vi "Main.vi"() -> ()   [LabVIEW 2014]
doc: "The Reaper Controller\n\nMarcin Twardak - twardakm@gmail.com\nLeszek Walulik\nJarosław Woźniak"
uses:
  Controls/Connection Configuration.ctl
  Controls/Controllers Clusters/Normal Operation Control Cluster.ctl
  Controls/Controllers.ctl
  Controls/Controllers Clusters/General Control Cluster.ctl
  Controls/Controllers Clusters/Game Pad Indicator Cluster.ctl
  Controls/Controllers Clusters/Game Pad Control Cluster.ctl
  Controls/Controllers Clusters/Mouse Control Cluster.ctl
  Controls/Queue Commands.ctl
  Controls/User Events Commands.ctl
  Controls/Connection Status.ctl
  Controls/User Help.ctl
  Controls/Configuration Files.ctl
  Controls/Simple Connection Settings Cluster.ctl
  <vilib>/Utility/miscctls.llb/LVBoundsTypeDef.ctl
  <vilib>/event_ctls.llb/usereventprio.ctl
  SubVIs/Convert From XML Configuration Files - Polymorphic/Simple Connection Settings Polymorphic.vi
  SubVIs/Convert From XML Configuration Files - Polymorphic/General Control Settings Polymporhic.vi
panel:
  in  "Normal Operation\nControl Cluster":T1 {"Game Pad Control Cluster"."Steering Wheel [Test]" scale=-100.0..100.0; "Game Pad Control Cluster"."Speed [Test]" scale=-100.0..100.0; "Game Pad Indicator Cluster"."Steering Wheel [%]" scale=-100.0..100.0; "Game Pad Indicator Cluster"."Speed" scale=0.0..100.0; "General Control Cluster"."Max Speed" max=100 step=5 scale=0.0..100.0}
  in  "Connection Conf\nCluster":T7
  out "User Help":string
  in  "Stop Button":bool
  # "THE REAPER"
  # "[Ctrl + Num] to switch"
  # "Mouse Controller"
  # "Game Pad Controller"
  # "Connection Configuration"
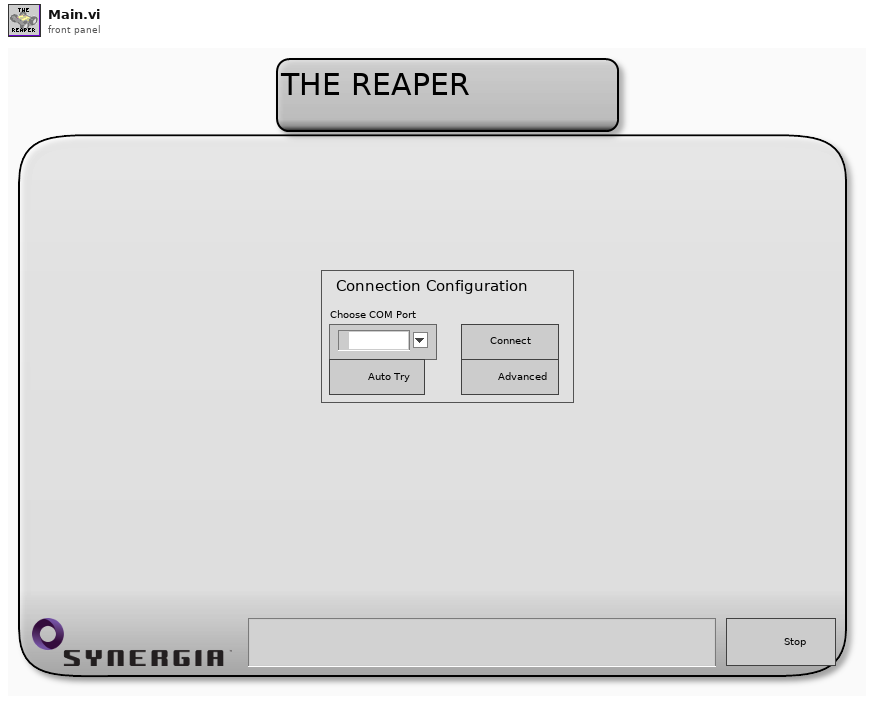
[diagram p1: front panel]
types:
  T1 = typedef "Normal Operation Control Cluster.ctl" = cluster{"Disconnect Button":bool, "Control Type":T2, "General Control Cluster":T3, "Game Pad Indicator Cluster":T4, "Game Pad Control Cluster":T5, "Mouse Control Cluster":T6}
  T2 = typedef "Controllers.ctl" = enum16{"Turned off", "Keyboard", "Mouse", "Pad", "Autonomous"}
  T3 = typedef "General Control Cluster.ctl" = cluster{"Max Speed":u8}
  T4 = typedef "Game Pad Indicator Cluster.ctl" = cluster{"Speed":u8, "Motor On?":bool, "Steering Wheel [%]":i8}
  T5 = typedef "Game Pad Control Cluster.ctl" = cluster{"Advanced Settings":bool, "Speed [Test]":i8, "Steering Wheel [Test]":i8, "Motor On [Test]":bool}
  T6 = typedef "Mouse Control Cluster.ctl" = cluster{"Mouse Controller":picture}
  T7 = typedef "Connection Configuration.ctl" = cluster{"Choose COM Port":refnum<visa-resource-name>, "Connect Button":bool, "Advanced Button":bool, "Auto Try Button":bool}
  T8 = typedef "Connection Status.ctl" = enum16{"Disconnected", "Connected"}
  T9 = typedef "User Events Commands.ctl" = enum16{"Consumer Error", "Stop App"}
  T10 = typedef "Queue Commands.ctl" = enum16{"Init", "Close App", "Producer Error", "Connect", "Try Auto Connect", "Is Connected?", "Advanced Connection Settings", "Disconnect", "Change Control Mode", "Stop Turn Off", "Start Turn Off", "Stop Keyboard", "Start Keyboard", "Stop Mouse", "Start Mouse", "Mouse", "Stop Pad", "Start Pad", "Pad", "Pad Advanced Settings", "Stop Autonomous", "Start Autonomous"}
  T11 = typedef "Configuration Files.ctl" = string
  T12 = typedef "Simple Connection Settings Cluster.ctl" = refnum<visa-resource-name>
  T13 = typedef "User Help.ctl" = enum16{"The Reaper Controller says hello!\nFirst you should establish connection with The Reaper.", "Connection established! Choose control mode.", "Something went wrong. Try another COM port.", "Disconnected. Do you want to connect again?", "Controls turned off", "Keyboard Mode", "Mouse Mode", "Pad Mode", "Autonomous Mode", "Unknown Operation occured", "Please connect before choosing control type!", "Settings available only if disconnected.", "Settings updated."}
  T14 = cluster{"Width":u16, "Style":enum32{"Solid", "Dash", "Dot", "DashDot", "DashDotDot"}}
  T15 = typedef "LVBoundsTypeDef.ctl" = cluster{"Width":u32, "Height":u32}
  T16 = typedef "usereventprio.ctl" = enum32{"high priority", "normal priority"}
  T17 = typedef "LVMouseTypeDef.ctl" = cluster{"Mouse Position":cluster{"X":i32, "Y":i32}, "Mouse Modifiers":cluster{"Button Down":bool, "Shift Mod":bool, "Menu Mod":bool, "Option Mod":bool}}
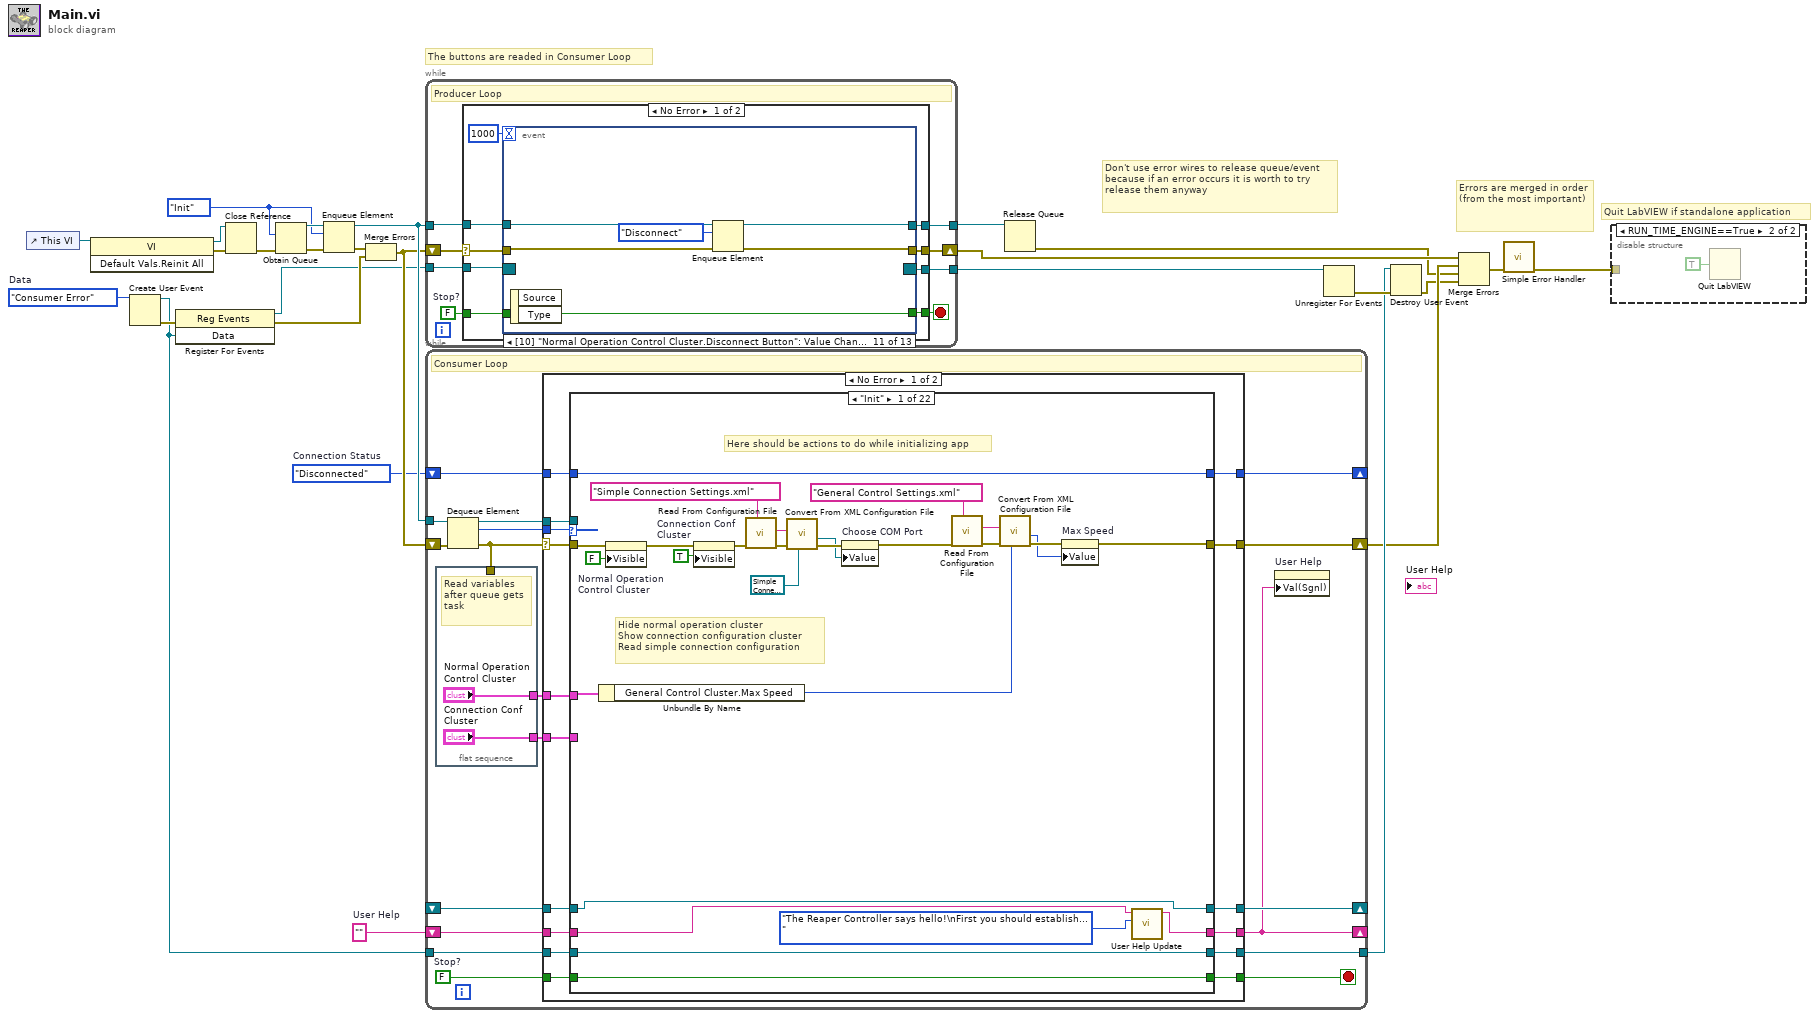
[diagram p0: block diagram]
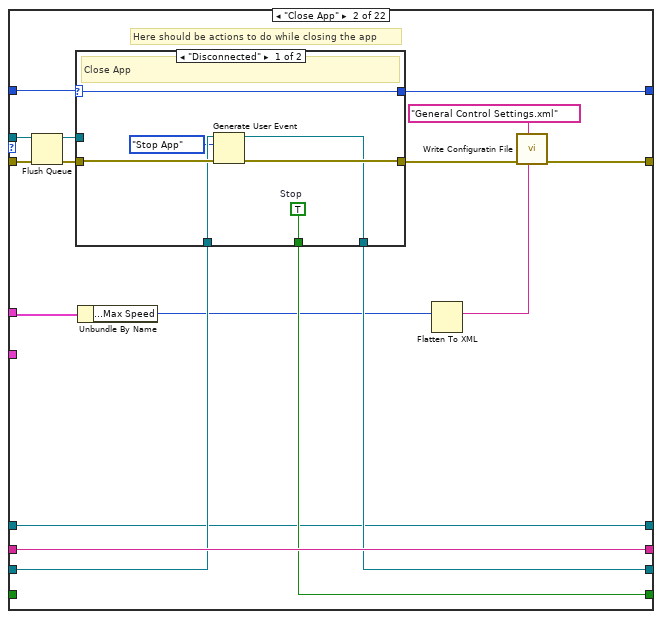
[diagram p3: hidden frame]
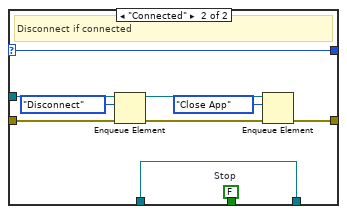
[diagram p4: hidden frame]
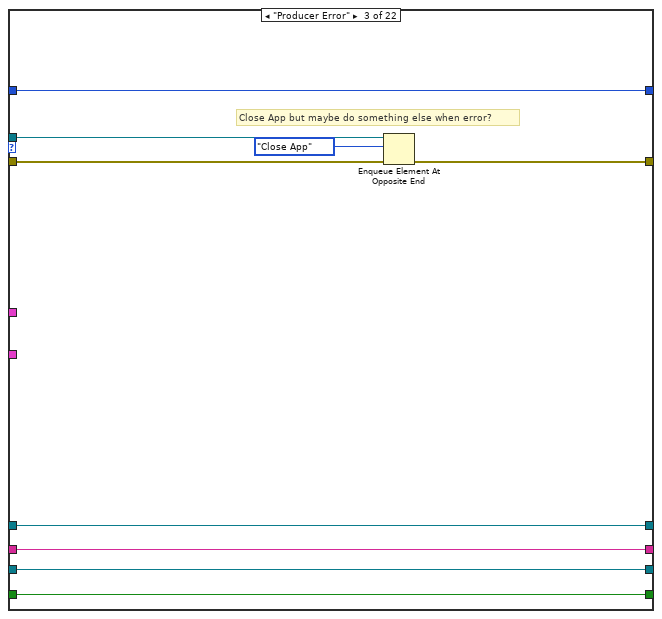
[diagram p5: hidden frame]
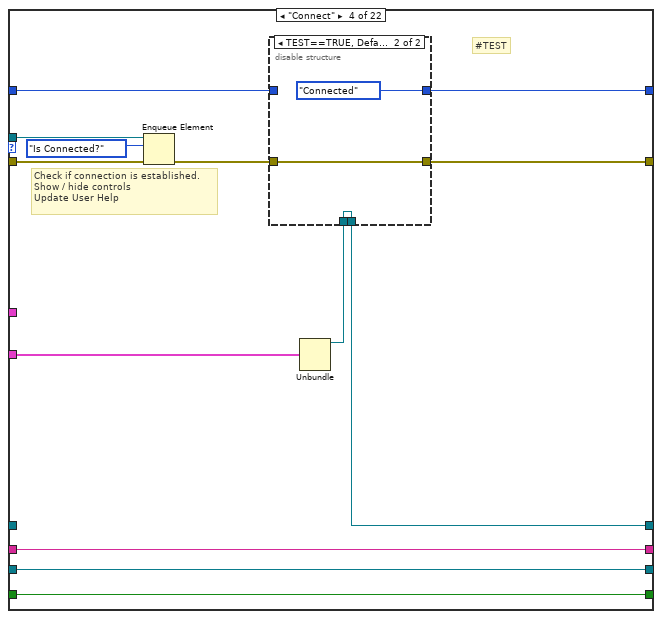
[diagram p6: hidden frame]
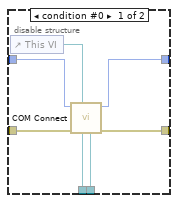
[diagram p7: hidden frame]
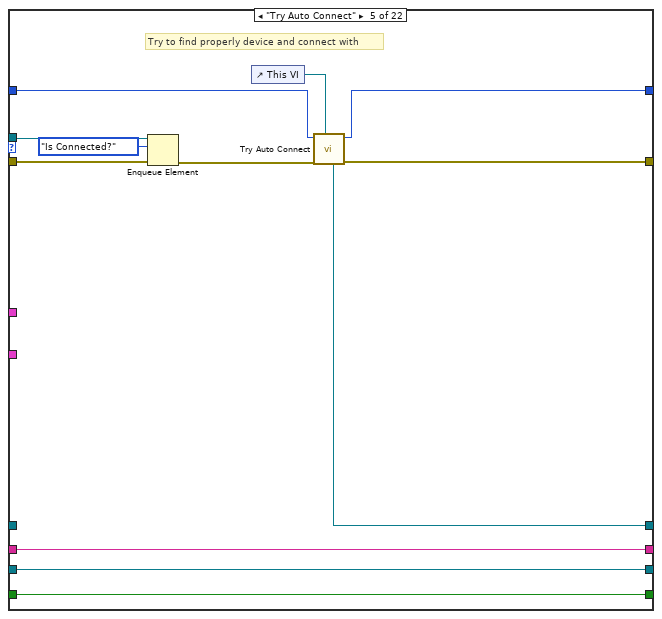
[diagram p8: hidden frame]
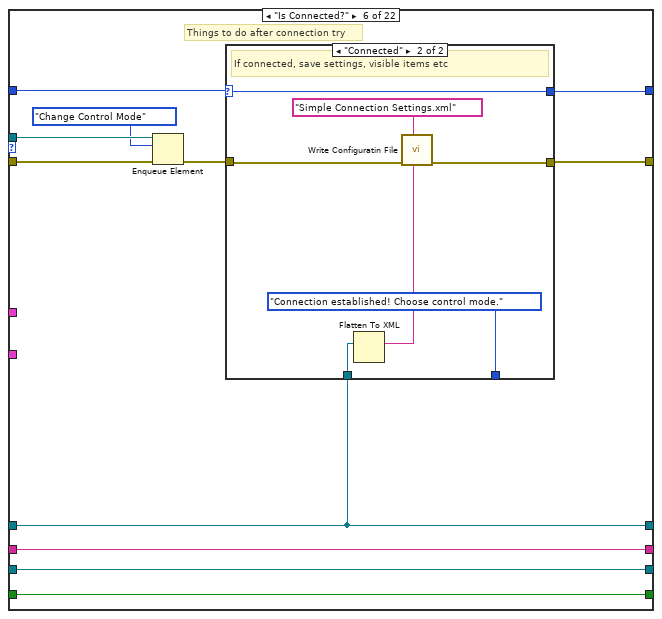
[diagram p9: hidden frame]
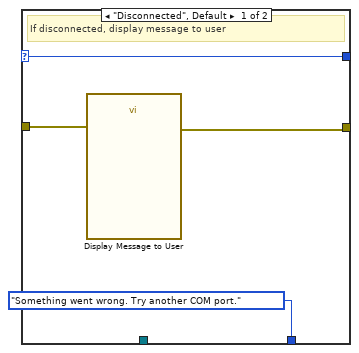
[diagram p10: hidden frame]
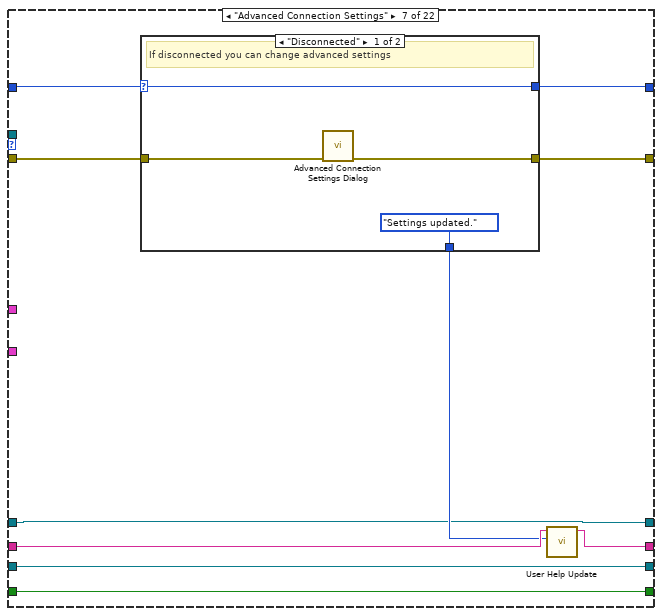
[diagram p11: hidden frame]
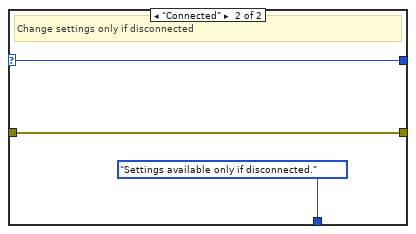
[diagram p12: hidden frame]
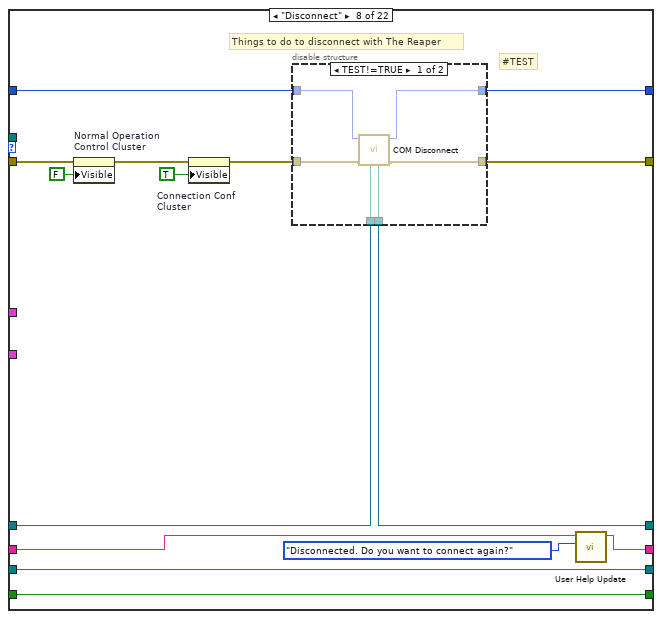
[diagram p13: hidden frame]
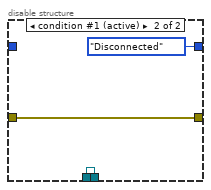
[diagram p14: hidden frame]
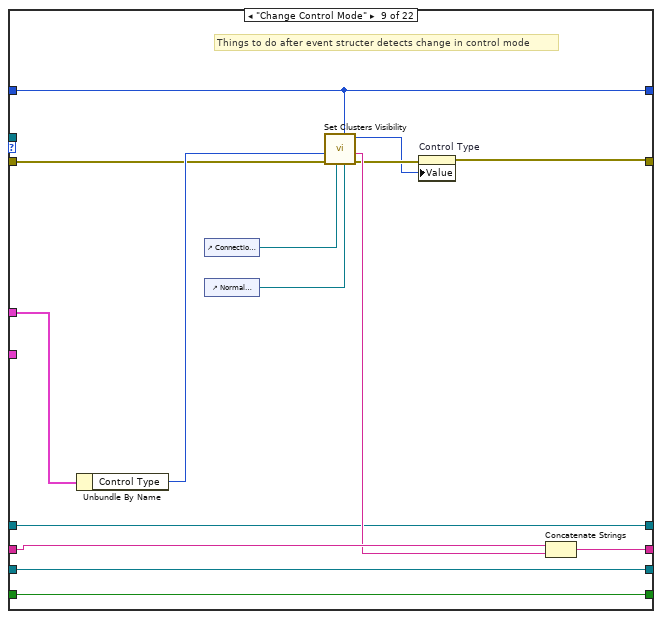
[diagram p15: hidden frame]
diagram:
  w1 = Connection_Status."Disconnected"  # Connection Status
  w3 = ""  # User Help
  w20 = User_Events_Commands."Consumer Error"  # Data
  w2 = Queue_Commands."Init"
  # "The buttons are readed in Consumer Loop"
  # "Quit LabVIEW if standalone application"
  # "Don't use error wires to release queue/event  because if an error occurs it is worth to try release them anyway"
  # "Errors are merged in order (from the most important)"
  n1 = control-ref of="This VI"() -> (w27:refnum<vi>)
  n2 = invoke class="VI" method="Default Vals.Reinit All"(reference=w27) -> (reference out=w25:refnum<vi>, error out=w26:errorcluster)  [unwired: 2 in, 1 out]
  n3 = Create User Event(user event datatype=w20) -> (user event=w14:refnum<user-event>, error out=w21:errorcluster)  [unwired: 1 in]
  n4 = register-events(error in=w21, w14) -> (reference out=w15:refnum<event-registration>, error out=w18:errorcluster)  [unwired: 1 in]
  n5 = Close Reference(reference=w25, error in (no error)=w26) -> (error out=w24:errorcluster)
  n6 = Obtain Queue(element data type=w2, error in (no error)=w24) -> (queue out=w22:refnum<queue>, error out=w23:errorcluster)  [unwired: 3 in, 1 out]
  n7 = Enqueue Element(queue=w22, element=w2, error in (no error)=w23) -> (queue out=w17:refnum<queue>, error out=w19:errorcluster)  [unwired: 1 in, 1 out]
  n8 = Merge Errors(w19, w18) -> (w16:errorcluster)
  n9 = while {
    tunnel: w17 -> [w34]
    shift-right: [w33] -> w9
    shift-left: w16 -> [w35]
    tunnel: w15 -> [w30]
    tunnel: [w29] -> w12
    tunnel: [w28] -> w13
    stop <- w32 stop-if-true
    w31 = FALSE  # Stop?
    # "Producer Loop"
    n10 = case shown="No Error" w35 {
      selector: w35 -> [w41 w176]
      tunnel: w34 -> [w42 w178]
      tunnel: [w40 w175] -> w33
      tunnel: [w37 w174] -> w32
      tunnel: w31 -> [w44 _]
      tunnel: w30 -> [w39 w173]
      tunnel: [w38 w173] -> w29
      tunnel: [w36 w172] -> w28
      frame No Error {
        n11 = event shown="[10] \"Normal Operation Control Cluster.Disconnect Button\": Value Change" {
          selector: w39 -> [_ _ _ _ _ _ _ _ _ _ _ _ _]
          dyn-events: [_ _ _ _ _ _ _ _ _ _ _ _ _] -> w38
          timeout: 1000 -> [_ _ _ _ _ _ _ _ _ _ _ _ _]
          tunnel: w44 -> [w46 _ _ w69 w98 w110 w116 w122 w128 w134 w140 w154 w170]
          tunnel: w42 -> [w45 w53 w58 w67 w96 w109 w115 w119 w127 w133 w139 w153 w169]
          tunnel: w41 -> [w47 w52 w56 w65 w94 w106 w112 w120 w124 w132 w137 w152 w167]
          tunnel: [w47 w51 w55 w64 w93 w105 w113 w121 w125 w131 w136 w144 w166] -> w40
          tunnel: [w46 w50 TRUE ("Stop") w69 w98 w110 w116 w122 w128 w134 w140 w154 w170] -> w37
          tunnel: [w45 w49 w57 w66 w95 w109 w114 w118 w126 w133 w138 w143 w168] -> w36
          event Timeout {
            n12 = event-data() -> ()  [unwired: 1 in, 1 out]
          }
          event "Stop Button": Value Change {
            w50 = FALSE  # Stop
            # "Don't stop\nStop due to User Event"
            n13 = event-data() -> ()  [unwired: 1 in, 1 out]
            n14 = Enqueue Element(queue=w53, element=Queue_Commands."Close App", error in (no error)=w52) -> (queue out=w49:refnum<queue>, error out=w51:errorcluster)  [unwired: 1 in, 1 out]
          }
          event User Event {
            # "User Event is used to catch consumer errors or stop prompt"
            n15 = event-data() -> ("Data"=w59:T9)  [unwired: 1 in]
            n16 = case shown="\"Stop App\"" w59 {
              tunnel: w58 -> [w61 w62]
              tunnel: [w61 w62] -> w57
              tunnel: w56 -> [w60 w63]
              tunnel: [w60 w63] -> w55
              frame "Consumer Error" {
              }
              frame "Stop App" {
              }
            }
          }
          event Menu Selection (User) {
            # "Shortcuts and menus undefined in LabVIEW"
            n17 = event-data() -> ("ItemTag"=w68:string)  [unwired: 1 in]
            n18 = case shown="\"Ctrl_3\"" w68 {
              tunnel: w67 -> [w71 w73 w79 w81 w85 w89]
              tunnel: [w71 w73 w79 w81 w85 w90] -> w66
              tunnel: [w70 w74 w77 w82 w86 w91] -> w64
              tunnel: w65 -> [w70 w75 w78 w83 w87 w92]
              frame Default {
              }
              frame "Ctrl_1" {
                # "Set Keyboard Mode"
                n19 = property on="Control Type" class="Enum (strict)"(error in=w75, "Val(Sgnl)"=Controllers."Keyboard" ("Value (Signaling)")) -> (error out=w74:errorcluster)  [unwired: 1 in, 1 out]
              }
              frame "Ctrl_2" {
                # "Set Mouse Mode"
                n20 = property on="Control Type" class="Enum (strict)"(error in=w78, "Val(Sgnl)"=Controllers."Mouse" ("Value (Signaling)")) -> (error out=w77:errorcluster)  [unwired: 1 in, 1 out]
              }
              frame "Ctrl_3" {
                # "Set Pad Mode"
                n21 = property on="Control Type" class="Enum (strict)"(error in=w83, "Val(Sgnl)"=Controllers."Pad" ("Value (Signaling)")) -> (error out=w82:errorcluster)  [unwired: 1 in, 1 out]
              }
              frame "Ctrl_4" {
                # "Set Autonomous Mode"
                n22 = property on="Control Type" class="Enum (strict)"(error in=w87, "Val(Sgnl)"=Controllers."Autonomous" ("Control Type")) -> (error out=w86:errorcluster)  [unwired: 1 in, 1 out]
              }
              frame "Advanced Settings" {
                # "Advanced Connection Settings"
                n23 = Enqueue Element(queue=w89, element=Queue_Commands."Advanced Connection Settings", error in (no error)=w92) -> (queue out=w90:refnum<queue>, error out=w91:errorcluster)  [unwired: 1 in, 1 out]
              }
            }
          }
          event Key Down {
            # "Other Key activities"
            n24 = event-data() -> ("Char"=w97:i16)  [unwired: 1 in]
            n25 = case shown="32" w97 {
              tunnel: w96 -> [w100 w104]
              tunnel: [w100 w104] -> w95
              tunnel: [w99 w102] -> w93
              tunnel: w94 -> [w99 w103]
              frame Default {
                # "Do nothing"
              }
              frame 32 {
                # "Spacebar - safety button"
                n26 = property on="Control Type" class="Enum (strict)"(error in=w103, "Val(Sgnl)"=Controllers."Turned off" ("Value (Signaling)")) -> (error out=w102:errorcluster)  [unwired: 1 in, 1 out]
              }
            }
          }
          event "User Help": Value Change {
            # "Scroll down"
            n27 = event-data() -> ()  [unwired: 1 in, 1 out]
            n28 = To Unsigned Long Integer(number=inf) -> (unsigned 32bit integer=w107:u32)
            n29 = property on="User Help" class="Str"(error in=w106, "Text.Scroll Position"=w107) -> (error out=w105:errorcluster)  [unwired: 1 in, 1 out]
          }
          event Value Change {
            n30 = event-data() -> ()  [unwired: 1 in, 1 out]
            n31 = Enqueue Element(queue=w115, element=Queue_Commands."Connect", error in (no error)=w112) -> (queue out=w114:refnum<queue>, error out=w113:errorcluster)  [unwired: 1 in, 1 out]
          }
          event Value Change {
            # "Tries to find all devices and connect with the good one"
            n32 = event-data() -> ()  [unwired: 1 in, 2 out]
            n33 = Enqueue Element(queue=w119, element=Queue_Commands."Try Auto Connect", error in (no error)=w120) -> (queue out=w118:refnum<queue>, error out=w121:errorcluster)  [unwired: 1 in, 1 out]
          }
          event Value Change {
            n34 = event-data() -> ()  [unwired: 1 in, 1 out]
            n35 = Enqueue Element(queue=w127, element=Queue_Commands."Advanced Connection Settings", error in (no error)=w124) -> (queue out=w126:refnum<queue>, error out=w125:errorcluster)  [unwired: 1 in, 1 out]
          }
          event Mouse Enter {
            # "If user pays attention to connection configuration stop blinking"
            n36 = event-data() -> ("CtlRef"=w130:refnum<vi>)  [unwired: 1 in]
            n37 = property class="Clust"(reference=w130, error in=w132, "Blinking"=FALSE) -> (error out=w131:errorcluster)  [unwired: 1 out]
          }
          event Value Change {
            n38 = event-data() -> ()  [unwired: 1 in, 2 out]
            n39 = Enqueue Element(queue=w139, element=Queue_Commands."Disconnect", error in (no error)=w137) -> (queue out=w138:refnum<queue>, error out=w136:errorcluster)  [unwired: 1 in, 1 out]
          }
          event Value Change {
            # "Do things to stop old control type and start the new one"
            n40 = event-data() -> ("NewVal"=w149:T2, "OldVal"=w150:T2)  [unwired: 1 in]
            n41 = case shown="\"Pad\"" w150 {
              tunnel: [Queue_Commands."Stop Turn Off" ("element") Queue_Commands."Stop Keyboard" ("element") Queue_Commands."Stop Mouse" ("element") Queue_Commands."Stop Pad" ("element") Queue_Commands."Stop Autonomous" ("element")] -> w146
              frame "Turned off" {
              }
              frame "Keyboard" {
              }
              frame "Mouse" {
              }
              frame "Pad" {
              }
              frame "Autonomous" {
              }
            }
            n42 = case shown="\"Pad\"" w149 {
              tunnel: [Queue_Commands."Start Turn Off" ("element") Queue_Commands."Start Keyboard" ("element") Queue_Commands."Start Mouse" ("element") Queue_Commands."Start Pad" ("element") Queue_Commands."Start Autonomous" ("element")] -> w141
              frame "Turned off" {
              }
              frame "Keyboard" {
              }
              frame "Mouse" {
              }
              frame "Pad" {
              }
              frame "Autonomous" {
              }
            }
            n43 = Enqueue Element(queue=w153, element=Queue_Commands."Change Control Mode", error in (no error)=w152) -> (queue out=w147:refnum<queue>, error out=w148:errorcluster)  [unwired: 1 in, 1 out]
            n44 = Enqueue Element(queue=w147, element=w146, error in (no error)=w148) -> (queue out=w142:refnum<queue>, error out=w145:errorcluster)  [unwired: 1 in, 1 out]
            n45 = Enqueue Element(queue=w142, element=w141, error in (no error)=w145) -> (queue out=w143:refnum<queue>, error out=w144:errorcluster)  [unwired: 1 in, 1 out]
          }
          event Value Change {
            n46 = event-data() -> ()  [unwired: 1 in, 1 out]
            n47 = Enqueue Element(queue=w169, element=Queue_Commands."Pad Advanced Settings", error in (no error)=w167) -> (queue out=w168:refnum<queue>, error out=w166:errorcluster)  [unwired: 1 in, 1 out]
          }
        }
      }
      frame Error {
        w174 = TRUE  # Stop
        # "If an error occurs send info as first element"
        n48 = Enqueue Element At Opposite End(queue=w178, element=Queue_Commands."Producer Error") -> (queue out=w172:refnum<queue>, error out=w177:errorcluster)  [unwired: 2 in, 1 out]
        n49 = Merge Errors(w177, w176) -> (w175:errorcluster)
      }
    }
  }
  n50 = while {
    tunnel: w17 -> [w184]
    shift-right: [w194] -> w8
    shift-left: w16 -> [w186]
    tunnel: w14 -> [w195]
    tunnel: [w193] -> w10
    shift-right: [w179] -> _
    shift-left: w3 -> [w191]
    shift-right: [w187] -> _
    shift-left: w1 -> [w188]
    shift-right: [w181] -> _
    shift-left: _ -> [w180]
    stop <- w192 stop-if-true
    w196 = FALSE  # Stop?
    # "Consumer Loop"
    n51 = flat-sequence {
      tunnel: ["Connection Conf\nCluster"] -> w190
      tunnel: ["Normal Operation\nControl Cluster"] -> w189
      tunnel: w182 -> [_]
      frame #0 {
        # "Read variables after queue gets task"
      }
    }
    n52 = Dequeue Element(queue=w184, error in (no error)=w186) -> (queue out=w185:refnum<queue>, element=w183:T10, error out=w182:errorcluster)  [unwired: 1 in, 1 out]
    n53 = case shown="No Error" w182 {
      selector: w182 -> [w203 w565]
      tunnel: w196 -> [w213 _]
      tunnel: w195 -> [w211 w568]
      tunnel: [w214 w563] -> w194
      tunnel: [w210 w562] -> w193
      tunnel: [w212 w561] -> w192
      tunnel: w191 -> [w209 w560]
      tunnel: [w208 w560] -> w179
      tunnel: w190 -> [w207 _]
      tunnel: w189 -> [w206 _]
      tunnel: w188 -> [w205 w559]
      tunnel: [w204 w559] -> w187
      tunnel: w185 -> [w202 _]
      tunnel: w183 -> [w201 _]
      tunnel: [w200 w558] -> w181
      tunnel: w180 -> [w199 w558]
      frame No Error {
        n54 = case shown="\"Init\"" w201 {
          tunnel: w202 -> [_ w257 w284 w286 w309 w321 _ _ _ _ _ _ _ _ w440 w479 _ w494 w527 _ _ _]
          tunnel: w203 -> [w233 w258 w283 w288 w311 w322 w344 w371 w383 w398 w404 w410 w416 w422 w441 w480 w487 w496 w528 w545 w546 w552]
          tunnel: [w215 w246 w282 w290 w316 w326 w343 w363 w386 w398 w404 w410 w416 w422 w434 w461 w487 w497 w519 w545 w546 w552] -> w214
          tunnel: w213 -> [w241 _ w281 w297 w319 w330 w351 w373 w397 w403 w409 w415 w421 w427 w446 w486 w492 w502 w533 w544 w551 w557]
          tunnel: [w241 w252 w281 w297 w319 w330 w351 w373 w397 w403 w409 w415 w421 w427 w446 w486 w492 w502 w533 w544 w551 w557] -> w212
          tunnel: w211 -> [w240 w250 w280 w296 w318 w329 w350 w372 w396 w402 w408 w414 w420 w426 w445 w485 w491 w501 w532 w543 w550 w556]
          tunnel: [w240 w249 w280 w296 w318 w329 w350 w372 w396 w402 w408 w414 w420 w426 w445 w485 w491 w501 w532 w543 w550 w556] -> w210
          tunnel: w209 -> [w235 w256 w279 w291 w317 w328 w347 w365 w389 w401 w407 w413 w419 w425 w444 w484 w490 w500 w531 w542 w549 w555]
          tunnel: [w237 w256 w279 w291 w317 w328 w346 w367 w390 w401 w407 w413 w419 w425 w444 w484 w490 w500 w531 w542 w549 w555] -> w208
          tunnel: w207 -> [_ _ _ w295 _ _ _ _ _ _ _ _ _ _ _ _ _ _ _ _ _ _]
          tunnel: w206 -> [w218 w244 _ _ _ _ _ _ w395 _ _ _ _ _ _ w456 _ _ w514 _ _ _]
          tunnel: w205 -> [w234 w253 w277 w294 w314 w325 w349 w362 w394 w400 w406 w412 w418 w424 w443 w483 w489 w499 w530 w541 w548 w554]
          tunnel: [w234 w251 w277 w289 w313 w327 w348 w361 w394 w400 w406 w412 w418 w424 w443 w483 w489 w499 w530 w541 w548 w554] -> w204
          tunnel: [w224 w248 w276 w292 w315 w324 w342 w359 w384 w399 w405 w411 w417 w423 w442 w482 w488 w498 w529 w540 w547 w553] -> w200
          tunnel: w199 -> [w224 w248 w276 _ _ w324 w342 w360 w384 w399 w405 w411 w417 w423 w442 w482 w488 w498 w529 w540 w547 w553]
          frame "Init" {
            # "Hide normal operation cluster\nShow connection configuration cluster\nRead simple connection configuration"
            # "Here should be actions to do while initializing app"
            n55 = Unbundle By Name(w218) -> ("General Control Cluster.Max Speed"=w217:u8)
            n56 = property on="Normal Operation\nControl Cluster" class="Clust"(error in=w233, "Visible"=FALSE) -> (error out=w230:errorcluster)  [unwired: 1 in, 1 out]
            n57 = property on="Connection Conf\nCluster" class="Clust"(error in=w230, "Visible"=TRUE) -> (error out=w231:errorcluster)  [unwired: 1 in, 1 out]
            n58 = call "Read From Configuration File.vi"("Settings"=T11 "Simple Connection Settings.xml", "error in (no error)"=w231) -> ("error out"=w228:errorcluster, "XML Elements"=w225:string)  [unwired: 8 in]
            n59 = call-poly "Convert From XML Configuration File.vi"("Simple Connection Settings"=T12 refnum ("VISA resource name"), "error in (no error)"=w228, "XML Elements"=w225) -> ("error out"=w227:errorcluster, "VISA resource name"=w226:T12)  [unwired: 7 in]
            n60 = property on="Choose COM Port" class="VISAName"(error in=w227, "Value"=w226) -> (error out=w223:errorcluster)  [unwired: 1 in, 1 out]
            n61 = call "Read From Configuration File.vi"("Settings"=T11 "General Control Settings.xml", "error in (no error)"=w223) -> ("error out"=w221:errorcluster, "XML Elements"=w220:string)  [unwired: 8 in]
            n62 = call-poly "Convert From XML Configuration File.vi"("Value"=w217, "error in (no error)"=w221, "XML Elements"=w220) -> ("error out"=w219:errorcluster, "Value Out"=w216:u8)  [unwired: 7 in]
            n63 = property on="Max Speed" class="Knob (strict)"(error in=w219, "Value"=w216) -> (error out=w215:errorcluster)  [unwired: 1 in, 1 out]
            n64 = call "User Help Update.vi"("Enum"=User_Help."The Reaper Controller says hello!\nFirst you should establish connection with The Reaper.", "User Help"=w235) -> ("User Help Out"=w237:string)  [unwired: 8 in, 1 out]
          }
          frame "Close App" {
            # "Here should be actions to do while closing the app"
            n65 = Flush Queue(queue=w257, error in (no error)=w258) -> (queue out=w254:refnum<queue>, error out=w255:errorcluster)  [unwired: 1 out]
            n66 = case shown="\"Disconnected\"" w253 {
              selector: w253 -> [w264 w269]
              tunnel: w255 -> [w263 w275]
              tunnel: w254 -> [_ w274]
              tunnel: [w262 w272] -> w247
              tunnel: [w265 w270] -> w252
              tunnel: [w264 w269] -> w251
              tunnel: w250 -> [w261 w266]
              tunnel: [w260 w266] -> w249
              frame "Disconnected" {
                w265 = TRUE  # Stop
                # "Close App"
                n67 = Generate User Event(user event=w261, event data cluster=User_Events_Commands."Stop App" ("event data"), error in=w263) -> (user event out=w260:refnum<user-event>, error out=w262:errorcluster)  [unwired: 1 in]
              }
              frame "Connected" {
                w270 = FALSE  # Stop
                # "Disconnect if connected"
                n68 = Enqueue Element(queue=w274, element=Queue_Commands."Disconnect", error in (no error)=w275) -> (queue out=w268:refnum<queue>, error out=w273:errorcluster)  [unwired: 1 in, 1 out]
                n69 = Enqueue Element(queue=w268, element=Queue_Commands."Close App", error in (no error)=w273) -> (error out=w272:errorcluster)  [unwired: 1 in, 2 out]
              }
            }
            n70 = Unbundle By Name(w244) -> ("General Control Cluster.Max Speed"=w243:u8)
            n71 = Flatten To XML(anything=w243) -> (xml string=w242:string)
            n72 = call "Write Configuratin File.vi"("XML String"=w242, "Settings"=T11 "General Control Settings.xml", "error in (no error)"=w247) -> ("error out"=w246:errorcluster)  [unwired: 8 in]
          }
          frame "Producer Error" {
            # "Close App but maybe do something else when error?"
            n73 = Enqueue Element At Opposite End(queue=w284, element=Queue_Commands."Close App", error in (no error)=w283) -> (error out=w282:errorcluster)  [unwired: 1 in, 2 out]
          }
          frame "Connect" {
            # "#TEST"
            # "Check if connection is established.\nShow / hide controls\nUpdate User Help"
            n74 = Enqueue Element(queue=w286, element=Queue_Commands."Is Connected?", error in (no error)=w288) -> (error out=w287:errorcluster)  [unwired: 1 in, 2 out]
            n75 = Unbundle(w295) -> ("Choose COM Port"=w293:refnum<visa-resource-name>)  [unwired: 3 out]
            n76 = disable-structure shown="TEST==TRUE, Default" {
              disable-tunnel: w287 -> [w304 w306]
              disable-tunnel: w294 -> [w303 _]
              disable-tunnel: w293 -> [w301 w307]
              disable-tunnel: [w300 w307] -> w292
              disable-tunnel: [w299 Connection_Status."Connected" ("Connection Status")] -> w289
              disable-tunnel: [w298 w306] -> w290
              frame condition #0 {
                n77 = control-ref of="This VI"() -> (w302:refnum<vi>)
                n78 = call "COM Connect.vi"("VISA resource name"=w301, "Main Front Panel Ref"=w302, "Error In"=w304, "Connection Status"=w303) -> ("Error Out"=w298:errorcluster, "Connection Status"=w299:T8, "VISA resource name OUT"=w300:refnum<visa-resource-name>)  [unwired: 5 in]
              }
              frame condition #1 (active) {
              }
            }
          }
          frame "Try Auto Connect" {
            # "Try to find properly device and connect with"
            n79 = Enqueue Element(queue=w309, element=Queue_Commands."Is Connected?", error in (no error)=w311) -> (error out=w310:errorcluster)  [unwired: 1 in, 2 out]
            n80 = control-ref of="This VI"() -> (w312:refnum<vi>)
            n81 = call "Try Auto Connect.vi"("Main VI"=w312, "Error In"=w310, "Connection Status"=w314) -> ("Error Out"=w316:errorcluster, "Connection Status Out"=w313:T8, "VISA resource name OUT"=w315:refnum<visa-resource-name>)  [unwired: 6 in]
          }
          frame "Is Connected?" {
            # "Things to do after connection try"
            n82 = Enqueue Element(queue=w321, element=Queue_Commands."Change Control Mode", error in (no error)=w322) -> (error out=w323:errorcluster)  [unwired: 1 in, 2 out]
            n83 = case shown="\"Connected\"" w325 {
              selector: w325 -> [w334 w339]
              tunnel: [w334 w339] -> w327
              tunnel: [w333 w338] -> w326
              tunnel: [User_Help."Something went wrong. Try another COM port." ("Enum") User_Help."Connection established! Choose control mode." ("Enum")] -> _
              tunnel: w323 -> [w331 w335]
              tunnel: w324 -> [_ w336]
              frame "Disconnected", Default {
                # "If disconnected, display message to user"
                n84 = call "Display Message to User"("error in (no error)"=w331) -> ("error out"=w333:errorcluster)  [unwired: 9 in, 1 out]
              }
              frame "Connected" {
                # "If connected, save settings, visible items etc"
                n85 = Flatten To XML(anything=w336) -> (xml string=w340:string)
                n86 = call "Write Configuratin File.vi"("XML String"=w340, "Settings"=T11 "Simple Connection Settings.xml", "error in (no error)"=w335) -> ("error out"=w338:errorcluster)  [unwired: 8 in]
              }
            }
          }
          frame "Advanced Connection Settings" {
            n87 = case shown="\"Disconnected\"" w349 {
              selector: w349 -> [w354 w358]
              tunnel: [w354 w358] -> w348
              tunnel: [User_Help."Settings updated." ("Enum") User_Help."Settings available only if disconnected." ("Enum")] -> w345
              tunnel: w344 -> [w353 w356]
              tunnel: [w352 w356] -> w343
              frame "Disconnected" {
                # "If disconnected you can change advanced settings"
                n88 = call "Advanced Connection Settings Dialog.vi"("Error In"=w353) -> ("Error Out"=w352:errorcluster)  [unwired: 10 in]
              }
              frame "Connected" {
                # "Change settings only if disconnected"
              }
            }
            n89 = call "User Help Update.vi"("Enum"=w345, "User Help"=w347) -> ("User Help Out"=w346:string)  [unwired: 8 in, 1 out]
          }
          frame "Disconnect" {
            # "#TEST"
            # "Things to do to disconnect with The Reaper"
            n90 = property on="Normal Operation\nControl Cluster" class="Clust"(error in=w371, "Visible"=FALSE) -> (error out=w370:errorcluster)  [unwired: 1 in, 1 out]
            n91 = property on="Connection Conf\nCluster" class="Clust"(error in=w370, "Visible"=TRUE) -> (error out=w364:errorcluster)  [unwired: 1 in, 1 out]
            n92 = disable-structure shown="TEST!=TRUE" {
              disable-tunnel: w364 -> [w379 w381]
              disable-tunnel: [w378 w381] -> w363
              disable-tunnel: w362 -> [w377 _]
              disable-tunnel: [w376 Connection_Status."Disconnected" ("Connection Status")] -> w361
              disable-tunnel: w360 -> [w375 w380]
              disable-tunnel: [w374 w380] -> w359
              frame condition #0 {
                n93 = call "COM Disconnect.vi"("VISA resource name"=w375, "Error In"=w379, "Connection Status"=w377) -> ("Error Out"=w378:errorcluster, "Connection Status"=w376:T8, "VISA resource name"=w374:refnum<visa-resource-name>)  [unwired: 6 in]
              }
              frame condition #1 (active) {
              }
            }
            n94 = call "User Help Update.vi"("Enum"=User_Help."Disconnected. Do you want to connect again?", "User Help"=w365) -> ("User Help Out"=w367:string)  [unwired: 8 in, 1 out]
          }
          frame "Change Control Mode" {
            # "Things to do after event structer detects change in control mode"
            n95 = Unbundle By Name(w395) -> ("Control Type"=w392:T2)
            n96 = control-ref of="Connection Conf\nCluster"() -> (w391:refnum<vi>)
            n97 = control-ref of="Normal Operation\nControl Cluster"() -> (w393:refnum<vi>)
            n98 = call "Set Clusters Visibility.vi"("Normal Operation Control Cluster"=w393, "Connection Status"=w394, "Connection Configuration Cluster"=w391, "Error In"=w383, "Control Type"=w392) -> ("Error Out"=w387:errorcluster, "User Help"=w388:string, "Control Type Out"=w385:T2)  [unwired: 4 in]
            n99 = property on="Control Type" class="Enum (strict)"(error in=w387, "Value"=w385) -> (error out=w386:errorcluster)  [unwired: 1 in, 1 out]
            n100 = Concatenate Strings(w389, w388) -> (w390:string)
          }
          frame "Stop Turn Off" {
            # "Things to do after changing control mode from Turn Off"
          }
          frame "Start Turn Off" {
            # "Things to do after changing control mode to Turn Off"
          }
          frame "Stop Keyboard" {
            # "Things to do after changing control mode from Keyboard"
          }
          frame "Start Keyboard" {
            # "Things to do after changing control mode to Keyboard"
          }
          frame "Stop Mouse" {
            # "Things to do after changing control mode from Mouse"
          }
          frame "Start Mouse" {
            # "Things to do after changing control mode to Mouse"
            n101 = Enqueue Element(queue=w440, element=Queue_Commands."Mouse", error in (no error)=w441) -> (error out=w438:errorcluster)  [unwired: 1 in, 2 out]
            n102 = property on="Mouse Controller" class="Pict"(error in=w438) -> ("Draw Area Size"=w437:T15)  [unwired: 1 in, 2 out]
            n103 = Divide(x=w437, y=T15 {"Width"=2, "Height"=2}) -> (x/y=w432:cluster{"Width":dbl, "Height":dbl})
            n104 = call <vilib>:"Draw Point.vi"("picture"=picture data[5B], "point(x,y)"=w432, "pen"=T14 {"Width"=4, "Style"=enum."Solid"}) -> ("new picture"=w431:picture)  [unwired: 6 in]
            n105 = for {
              N: 8 -> [_]
              tunnel: w432 -> [w453]
              shift-right: [w449] -> w430
              shift-left: w431 -> [w450]
              tunnel: T14 {"Width"=1, "Style"=enum."Dash"} ("pen") -> [w447]
              i -> [w454]
              n106 = Increment(x=w454) -> (x+1=w452:i32)
              n107 = Multiply(x=40, y=w452) -> (x*y=w448:i32)
              n108 = call <vilib>:"Draw Circle by Radius.vi"("pen"=w447, "pixel center"=w453, "radius"=w448, "picture"=w450) -> ("new picture"=w449:picture)  [unwired: 7 in]
            }
            n109 = property on="Mouse Controller" class="Pict"("Value"=w430) -> (error out=w434:errorcluster)  [unwired: 2 in, 1 out]
          }
          frame "Mouse" {
            n110 = Unbundle By Name(w456) -> ("General Control Cluster.Max Speed"=w455:u8)
            n111 = Enqueue Element(queue=w479, element=Queue_Commands."Mouse", error in (no error)=w480) -> (error out=w477:errorcluster)  [unwired: 1 in, 2 out]
            n112 = property on="Mouse Controller" class="Pict"(error in=w477) -> (error out=w460:errorcluster, "Mouse"=w476:T17, "Width"=w474:u32, "Height"=w470:u32)  [unwired: 1 in, 1 out]
            n113 = To Double Precision Float(number=w474) -> (double precision float=w475:dbl)
            n114 = To Double Precision Float(number=w470) -> (double precision float=w471:dbl)
            n115 = Unbundle By Name(w476) -> ("Mouse Modifiers.Button Down"=w459:bool, "Mouse Position.X"=w469:i32, "Mouse Position.Y"=w468:i32)
            n116 = Divide(x=w475, y=100.0) -> (x/y=w466:dbl)
            n117 = Divide(x=w471, y=100.0) -> (x/y=w464:dbl)
            n118 = To Double Precision Float(number=w469) -> (double precision float=w467:dbl)
            n119 = To Double Precision Float(number=w468) -> (double precision float=w465:dbl)
            n120 = Divide(x=w467, y=w466) -> (x/y=w463:dbl)
            n121 = Divide(x=w465, y=w464) -> (x/y=w462:dbl)
            n122 = To Byte Integer(number=w463) -> (8bit integer=w458:i8)
            n123 = To Byte Integer(number=w462) -> (8bit integer=w457:i8)
            n124 = call "Generate Control Command.vi"("Maximum Speed"=w455, "Error In"=w460, "Motor On"=w459, "Steering wheel"=w458, "Speed"=w457) -> ("Error Out"=w461:errorcluster)  [unwired: 4 in, 2 out]
            n125 = Wait Until Next ms Multiple(millisecond multiple=u32 20) -> ()  [unwired: 1 out]
          }
          frame "Stop Pad" {
            # "Things to do after changing control mode from Game Pad"
          }
          frame "Start Pad" {
            # "#TEST"
            # "Things to do after changing control mode to Pad"
            n126 = Enqueue Element(queue=w494, element=Queue_Commands."Pad", error in (no error)=w496) -> (error out=w495:errorcluster)  [unwired: 1 in, 2 out]
            n127 = disable-structure shown="TEST==TRUE, Default" {
              disable-tunnel: w495 -> [w507 w512]
              disable-tunnel: [w504 w509] -> w497
              frame condition #0 {
                w503 = FALSE
                # "Make unvisible test controls if normal operation"
                n128 = property on="Motor On [Test]" class="Bool (strict)"(error in=w507, "Visible"=w503) -> (error out=w506:errorcluster)  [unwired: 1 in, 1 out]
                n129 = property on="Speed [Test]" class="Slide (strict)"(error in=w506, "Visible"=w503) -> (error out=w505:errorcluster)  [unwired: 1 in, 1 out]
                n130 = property on="Steering Wheel [Test]" class="Slide (strict)"(error in=w505, "Visible"=w503) -> (error out=w504:errorcluster)  [unwired: 1 in, 1 out]
              }
              frame condition #1 (active) {
                w508 = TRUE
                # "Make visible test controls if test"
                n131 = property on="Motor On [Test]" class="Bool (strict)"(error in=w512, "Visible"=w508) -> (error out=w511:errorcluster)  [unwired: 1 in, 1 out]
                n132 = property on="Speed [Test]" class="Slide (strict)"(error in=w511, "Visible"=w508) -> (error out=w510:errorcluster)  [unwired: 1 in, 1 out]
                n133 = property on="Steering Wheel [Test]" class="Slide (strict)"(error in=w510, "Visible"=w508) -> (error out=w509:errorcluster)  [unwired: 1 in, 1 out]
              }
            }
          }
          frame "Pad" {
            # "#TEST"
            n134 = Enqueue Element(queue=w527, element=Queue_Commands."Pad", error in (no error)=w528) -> (error out=w524:errorcluster)  [unwired: 1 in, 2 out]
            n135 = Unbundle By Name(w514) -> ("General Control Cluster.Max Speed"=w513:u8)
            n136 = disable-structure shown="TEST==TRUE, Default" {
              disable-tunnel: w524 -> [w534 w539]
              disable-tunnel: [w534 w539] -> w523
              disable-tunnel: w514 -> [_ w538]
              disable-tunnel: [_ w537] -> w517
              disable-tunnel: [_ w536] -> w516
              disable-tunnel: [_ w535] -> w515
              frame condition #0 {
                # "Here should be readed information from joystick"
              }
              frame condition #1 (active) {
                n137 = Unbundle By Name(w538) -> ("Game Pad Control Cluster.Speed [Test]"=w537:i8, "Game Pad Control Cluster.Steering Wheel [Test]"=w536:i8, "Game Pad Control Cluster.Motor On [Test]"=w535:bool)
              }
            }
            n138 = Absolute Value(x=w517) -> (abs(x)=w518:i8)
            n139 = property on="Speed" class="Knob (strict)"(error in=w523, "Value"=w518) -> (error out=w522:errorcluster)  [unwired: 1 in, 1 out]
            n140 = property on="Steering Wheel [%]" class="Slide (strict)"(error in=w522, "Value"=w516) -> (error out=w521:errorcluster)  [unwired: 1 in, 1 out]
            n141 = property on="Motor On?" class="Bool (strict)"(error in=w521, "Val(Sgnl)"=w515) -> (error out=w520:errorcluster)  [unwired: 1 in, 1 out]
            n142 = call "Generate Control Command.vi"("Maximum Speed"=w513, "Error In"=w520, "Motor On"=w515, "Steering wheel"=w516, "Speed"=w517) -> ("Error Out"=w519:errorcluster)  [unwired: 4 in, 2 out]
            n143 = Wait Until Next ms Multiple(millisecond multiple=u32 20) -> ()  [unwired: 1 out]
          }
          frame "Pad Advanced Settings" {
            # "Opens Pad advanced settings window"
          }
          frame "Stop Autonomous" {
            # "Things to do after changing control mode from Autonomous"
          }
          frame "Start Autonomous" {
            # "Things to do after changing control mode to Autonomous"
          }
        }
      }
      frame Error {
        w561 = TRUE  # Stop
        # "If an error occurs generate event -> Producer Loop need to be stopped"
        n144 = Generate User Event(priority (normal)=usereventprio."high priority", user event=w568, event data cluster=User_Events_Commands."Consumer Error" ("event data")) -> (user event out=w562:refnum<user-event>, error out=w564:errorcluster)  [unwired: 1 in]
        n145 = Merge Errors(w565, w564) -> (w563:errorcluster)
      }
    }
    n146 = property on="User Help" class="Str"("Val(Sgnl)"=w179) -> ()  [unwired: 2 in, 2 out]
  }
  n147 = Release Queue(queue=w13) -> (error out=w7:errorcluster)  [unwired: 2 in, 2 out]
  n148 = Unregister For Events(event registration refnum=w12) -> (error out=w11:errorcluster)  [unwired: 1 in]
  n149 = Destroy User Event(user event=w10, error in=w11) -> (error out=w6:errorcluster)
  n150 = Merge Errors(w9, w8, w7, w6) -> (w5:errorcluster)
  n151 = call <vilib>:"Simple Error Handler.vi"("error in (no error)"=w5) -> ("error out"=w4:errorcluster)  [unwired: 4 in, 4 out]
  n152 = disable-structure shown="RUN_TIME_ENGINE==True" {
    disable-tunnel: w4 -> [_ _]
    frame condition #0 (active) {
    }
    frame condition #1 {
      n153 = Quit LabVIEW(quit? (T)=TRUE) -> ()
    }
  }
